vi "tank.vi"() -> ()   [LabVIEW 2024]
uses:
  Control 1.ctl
panel:
  in  "Empty/Fill":bool
  out "Empting Pump":bool
  out "Filling Pump":bool
  in  "Tank Level":T1 scale=0.0..100.0
  in  "Low Limit":dbl
  in  "High Limit":dbl
  out "Tank":dbl(slide) scale=0.0..10.0
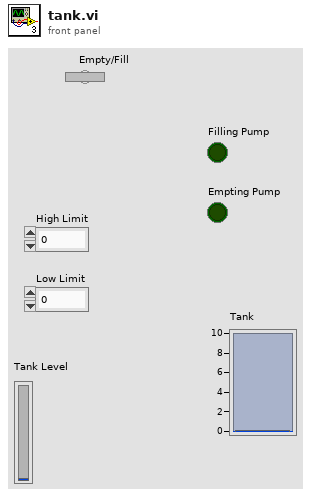
[diagram p1: front panel]
types:
  T1 = typedef "Control 1.ctl" = u8
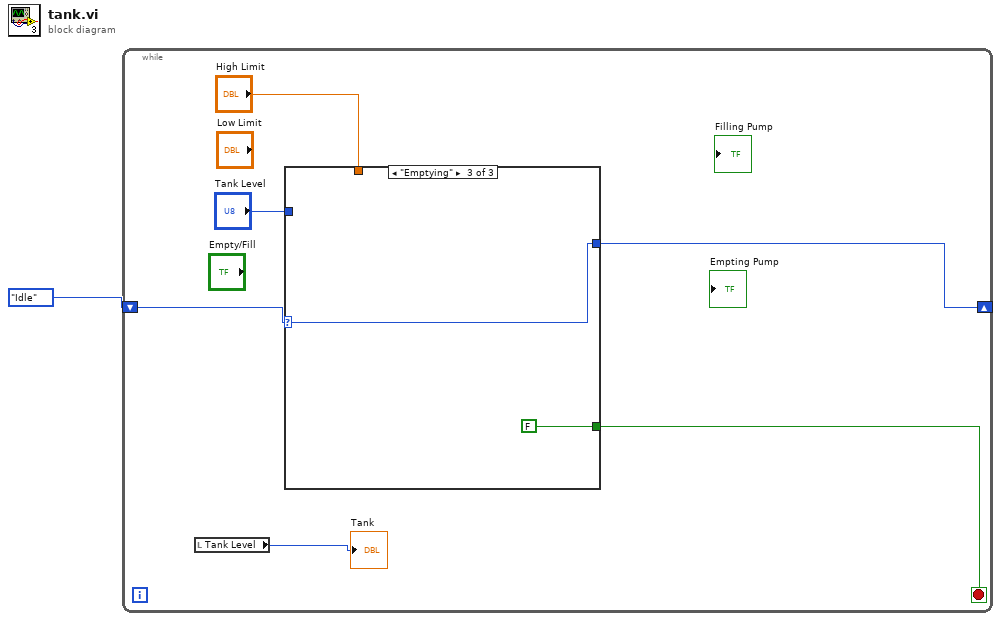
[diagram p0: block diagram]
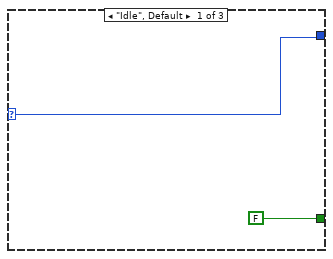
[diagram p2: hidden frame]
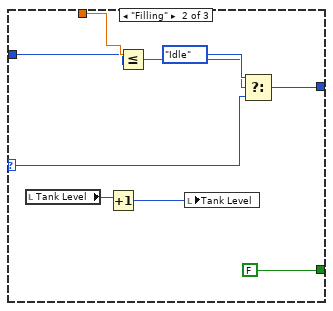
[diagram p3: hidden frame]
diagram:
  n1 = while {
    shift-right: [w2] -> _
    shift-left: enum16{"Idle", "Filling", "Emptying"}."Idle" -> [w7]
    stop <- w6 stop-if-true
    n2 = local read "Tank Level"() -> (→"Tank":T1)
    n3 = case shown="\"Emptying\"" w7 {
      selector: w7 -> [w8 w11 w19]
      tunnel: [FALSE FALSE FALSE] -> w6
      tunnel: "High Limit" -> [_ w15 _]
      tunnel: "Tank Level" -> [_ w14 _]
      tunnel: [w8 w10 w19] -> w2
      frame "Idle", Default {
      }
      frame "Filling" {
        n4 = local read "Tank Level"() -> (w16:T1)
        n5 = Increment(x=w16) -> (x+1=w17:T1)
        n6 = Less Or Equal?(x=w15, y=w14) -> (x <= y?=w12:bool)
        n7 = local write "Tank Level"(w17) -> ()
        n8 = Select(t=enum16{"Idle", "Filling", "Emptying"}."Idle", s=w12, f=w11) -> (s? t:f=w10:enum16{"Idle", "Filling", "Emptying"})
      }
      frame "Emptying" {
      }
    }
  }
